vi "Run Memory Test.vi"(8 "error in (no error)":errorcluster, 10 "Position":u32, 11 "MTS Memory Test in":refnum<class "MTS Memory Test.lvclass">) -> (0 "error out":errorcluster, 3 "Test Passed":bool)   [LabVIEW 2015, in "MTS Memory Test.lvclass"]
doc: "Performs the memory test using an MTS class object."
uses:
  MTS Memory Test.lvclass
  Classes/Manufacturing Test/Class/SC Manufacturing Test.lvclass
  <vilib>/Cree, Inc/Cree Test Framework/Classes/Base Objects/Base Class/Base Class/Base Class.lvclass
  Common RF Tests/RF Common Tests.lvclass
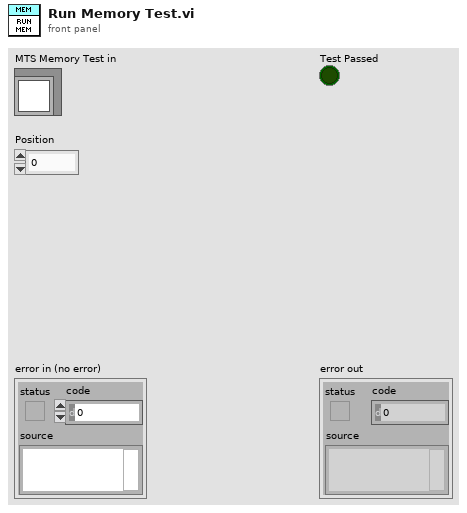
[diagram p1: front panel]
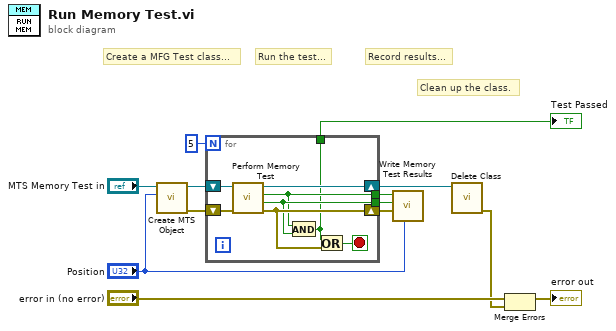
[diagram p0: block diagram]
diagram:
  # "Clean up the class."
  # "Record results..."
  # "Run the test..."
  # "Create a MFG Test class..."
  n1 = call "Create MTS Object.vi"("Position"="Position", "RF Common Tests in"="MTS Memory Test in") -> ("error out"=w8:errorcluster, "SC Manufacturing Test out"=w9:refnum<class "SC Manufacturing Test.lvclass">)  [unwired: 8 in]
  n2 = for {
    N: 5 -> [_]
    shift-right: [w21] -> w5
    shift-left: w9 -> [w20]
    shift-right: [w17] -> w1
    shift-left: w8 -> [w19]
    tunnel: [w16] -> w11
    tunnel: [w15] -> w3
    tunnel: [w14] -> w6
    stop <- w18 stop-if-true
    n3 = call "Perform Memory Test.vi"("error in (no error)"=w19, "Acrobat Template in"=w20) -> ("error out"=w17:errorcluster, "Read Passed"=w16:bool, "Write Passed"=w15:bool, "Acrobat Template out"=w21:refnum<class "SC Manufacturing Test.lvclass">)  [unwired: 6 in]
    n4 = And(x=w15, y=w16) -> (x .and. y?=w14:bool)
    n5 = Or(x=w14, y=w17) -> (x .or. y?=w18:bool)
  }
  "Test Passed" <- w6
  n6 = call "Write Memory Test Results.vi"("Position"="Position", "error in (no error)"=w1, "Read Passed"=w11, "Write Passed"=w3) -> ()  [unwired: 8 in]
  n7 = call <vilib>:"Delete Class.vi"("Base Class in"=w5) -> ("error out"=w4:errorcluster)  [unwired: 9 in, 1 out]
  n8 = Merge Errors("error in (no error)", w4) -> (→"error out":errorcluster)
